vi "Split_string_token--untested.vi"(7 "Ignore case (TRUE def)":bool=TRUE, 10 "Token":string="\\", 11 "Input String":string="c:\\DATA\\20141011-102717-0.fits") -> (1 "Strings positions":i32[](array[numeric])=[2, 4], 2 "Array Length":i32=2, 3 "Array":string[](array[string])=["DATA\\20141011-102717-0.FITS", "20141011-102717-0.FITS"])   [LabVIEW 2012]
panel:
  out "String Array Selected":string[](array[string])=["c:\\DATA\\20141011-102717-0.fits", "c:\\DATA\\20141011-102717-1.fits"]
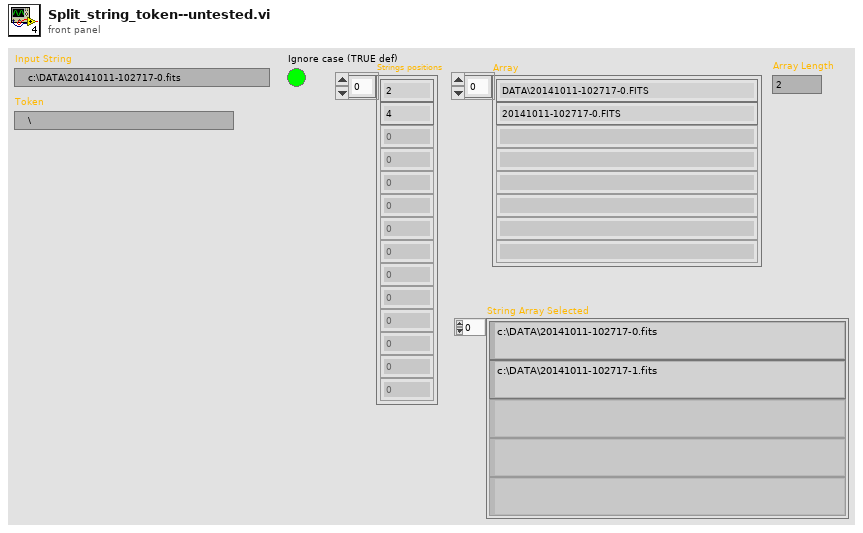
[diagram p1: front panel]
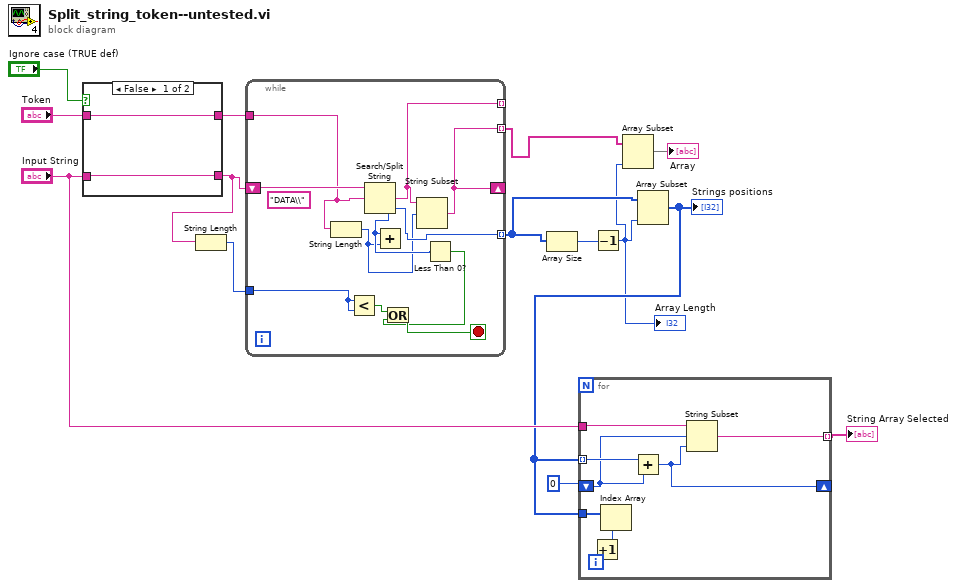
[diagram p0: block diagram]
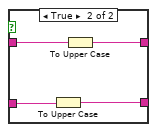
[diagram p2: hidden frame]
diagram:
  n1 = case shown="False" "Ignore case (TRUE def)" {
    tunnel: [w15 w20] -> w14
    tunnel: "Input String" -> [w15 w19]
    tunnel: "Token" -> [w16 w18]
    tunnel: [w16 w17] -> w10
    frame False {
    }
    frame True {
      n2 = To Upper Case(1:w19) -> (0:w20:string)
      n3 = To Upper Case(1:w18) -> (0:w17:string)
    }
  }
  n4 = String Length(string=w14) -> (length=w13:i32)
  n5 = while {
    shift-right: [w27] -> _
    shift-left: w14 -> [w28]
    tunnel: [w27] -> w9 mode=indexing
    tunnel: w13 -> [w25]
    tunnel: [w24] -> w7 mode=indexing
    tunnel: [w22] -> _ mode=indexing
    tunnel: w10 -> [w21]
    stop <- w29 stop-if-true
    (unwired) "DATA\\" ("search string/char (-)")
    n6 = String Length(string=w21) -> (length=w23:i32)
    n7 = Less?(x=w25, y=w25) -> (x < y?=w30:bool)
    n8 = Search/Split String(string=w28, search string/char (-)=w21) -> (match + rest of string=w22:string, offset of match=w24:i32)  [unwired: 1 in, 1 out]
    n9 = Add(x=w24, y=w23) -> ()  [unwired: 1 out]
    n10 = String Subset(string=w22, offset (0)=w23) -> (substring=w27:string)  [unwired: 1 in]
    n11 = Less Than 0?(x=w24) -> (x < 0?=w26:bool)
    n12 = Or(x=w30, y=w26) -> (x .or. y?=w29:bool)
  }
  n13 = Array Size(array=w7) -> (size(s)=w8:i32)
  n14 = Decrement(x=w8) -> (x-1=w1:i32)
  "Array Length" <- w1
  n15 = Array Subset(array=w9, length=w1) -> (→"Array":string[])  [unwired: 1 in]
  n16 = Array Subset(array=w7, length=w1) -> (w3:i32[])  [unwired: 1 in]
  "Strings positions" <- w3
  n17 = for {
    tunnel: "Input String" -> [w38]
    tunnel: w3 -> [w37] mode=indexing
    shift-right: [w32] -> _
    shift-left: 0 -> [w31]
    tunnel: w3 -> [w35]
    tunnel: [w33] -> w2 mode=indexing
    i -> [w36]
    n18 = Increment(x=w36) -> (x+1=w34:i32)
    n19 = Index Array(array=w35, index=w34) -> ()  [unwired: 1 out]
    n20 = Add(x=w37, y=w31) -> (x+y=w32:i32)
    n21 = String Subset(string=w38, offset (0)=w31, length (rest)=w32) -> (substring=w33:string)
  }
  "String Array Selected" <- w2
